vi "GetFullName.vi"(8 "error in (no error)":errorcluster, 11 "DocumentClass in":refnum<class "Characteristic.lvclass">) -> (0 "error out":errorcluster, 2 "FileName":string, 3 "DocumentClass out":refnum<class "Characteristic.lvclass">)   [LabVIEW 2021, in "ProligentXMLGenerator.lvlib" / "Characteristic.lvclass"]
doc: "Get Full Name\n\nCharacteristics are unique among siblings by their FullName property.\n\nIt's limited to 434 characters."
uses:
  Characteristic.lvclass
  Characteristic.lvclass/Characteristic.ctl
  Base/NonEmptyString_434/NonEmptyString_434.lvclass
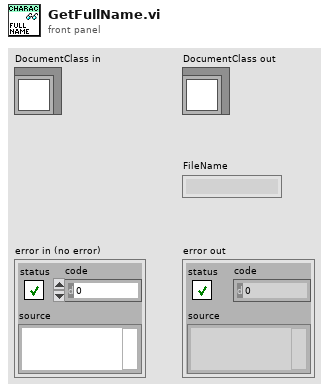
[diagram p1: front panel]
types:
  T1 = typedef "ProligentXMLGenerator.lvlib/Characteristic.lvclass/Data.ctl" = cluster{"Name":string, "CustomData":refnum<class "CustomData.lvclass">, "FullName":refnum<class "NonEmptyString_434.lvclass">, "Value":refnum<class "String_2000.lvclass">}
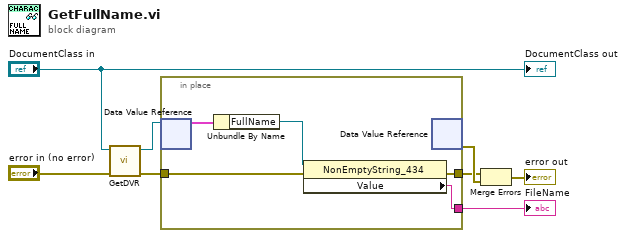
[diagram p0: block diagram]
diagram:
  n1 = call "GetDVR.vi"("error in"="error in (no error)", "Document in"="DocumentClass in") -> ("error out"=w5:errorcluster, "DVRReference"=w7:refnum<data-value>)  [unwired: 8 in]
  n2 = in-place "In Place Element Structure" {
    in-place-border: [w10] -> w6
    in-place-border: w5 -> [w11]
    in-place-border: [w9] -> w4
    n3 = in-place-dvr #1(w7) -> (w13:T1)  [unwired: 1 out]
    n4 = Unbundle By Name(w13) -> ("FullName"=w12:refnum<class "NonEmptyString_434.lvclass">)
    n5 = property on="Property Node" class="NonEmptyString_434"(reference=w12, error in=w11) -> (error out=w9:errorcluster, "Value"=w10:string)  [unwired: 1 out]
    n6 = in-place-dvr #1() -> (w8:errorcluster)  [unwired: 1 in, 1 out]
  }
  "FileName" <- w6
  n7 = Merge Errors(w4, w8) -> (→"error out":errorcluster)
  "DocumentClass out" <- "DocumentClass in"
